vi "Memory.Pointer.Read.Safe.1D.U8.vi"(8 "error in (no error)":errorcluster, 9 "count":u64 format="%d elements", 10 "buffer in":u8[](array[numeric]), 11 "pointer in":refnum<class "Memory.Pointer.lvclass">) -> (0 "error out":errorcluster, 1 "count out":u64 format="%d elements", 2 "buffer out":u8[](array[numeric]), 3 "pointer out":refnum<class "Memory.Pointer.lvclass">)   [LabVIEW 2016, in "Memory Manager.lvlib" / "Memory.Pointer.lvclass"]
doc: "Reads from the address specified by <b>pointer</b> into <b>value</b>.\n\n<b>Note:</b> This VI is <b>safe</b>.\n\nSafe means that this function evaluates the size parameter of <b>pointer</b> to ensure that is inbounds of allocated memory before peforming a memory read/write. Reading/writing more data to a pointer than it has allocated can corrupt or crash LabVIEW."
uses:
  Memory.Pointer.lvclass
  Memory.Pointer.lvclass/Memory.Pointer.ctl
  Accessors/Get Address.vi
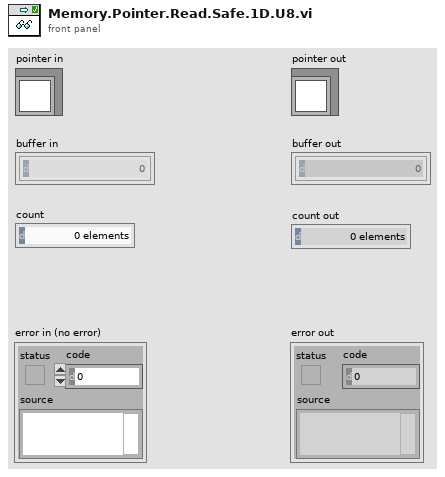
[diagram p1: front panel]
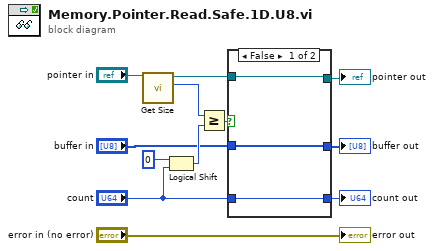
[diagram p0: block diagram]
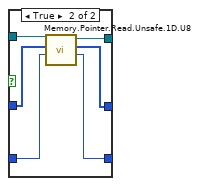
[diagram p2: hidden frame]
diagram:
  n1 = call "Get Size.vi"("Pointer in"="pointer in") -> ("size"=w10:u64, "Pointer out"=w8:refnum<class "Memory.Pointer.lvclass">)  [unwired: 8 in, 1 out]
  n2 = Logical Shift(y=i16 0, x="count") -> (x << y=w9:u64)
  n3 = Greater Or Equal?(x=w10, y=w9) -> (x >= y?=w1:bool)
  n4 = case shown="False" w1 {
    tunnel: w8 -> [w15 w21]
    tunnel: [w15 w20] -> w7
    tunnel: "buffer in" -> [w14 w19]
    tunnel: [w14 w18] -> w5
    tunnel: "count" -> [w13 w17]
    tunnel: [w13 w16] -> w3
    frame False {
    }
    frame True {
      n5 = call "Memory.Pointer.Read.Unsafe.1D.U8.vi"("count"=w17, "buffer in"=w19, "pointer in"=w21) -> ("count out"=w16:u64, "buffer out"=w18:u8[], "pointer out"=w20:refnum<class "Memory.Pointer.lvclass">)  [unwired: 5 in, 1 out]
    }
  }
  "pointer out" <- w7
  "buffer out" <- w5
  "count out" <- w3
  "error out" <- "error in (no error)"
